vi "Bench_Tests.vi"() -> ()   [LabVIEW 2026]
panel:
  out "cell sum":dbl
  out "limits ok?":bool
  out "results":T1(array[cluster])
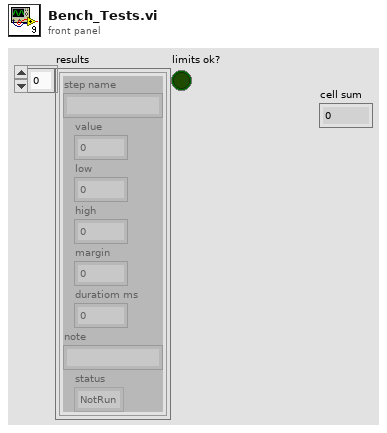
[diagram p1: front panel]
types:
  T1 = cluster{"step name":string, "value":dbl, "low":dbl, "high ":dbl, "margin":dbl, "duratiom ms":dbl, "note":string, "status":enum16{"NotRun", "Pass", "Fail", "Skipped"}}[]
  T2 = cluster{"iso low":dbl, "iso high":dbl, "cell low":dbl, "cell high":dbl, "dv low":dbl, "dv high":dbl, "pack low":dbl, "pack high":dbl}
  T3 = cluster{"step name":string, "value":dbl, "low":dbl, "high ":dbl, "margin":dbl, "duration ms":dbl, "note":string, "status":enum16{"NotRun", "Pass", "Fail", "Skipped"}}[]
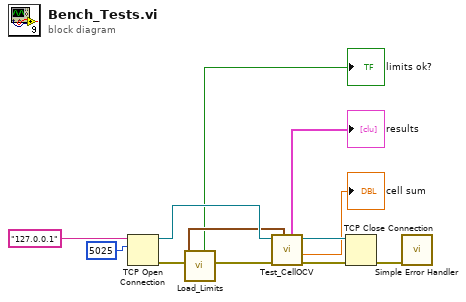
[diagram p0: block diagram]
diagram:
  n1 = TCP Open Connection(address="127.0.0.1", remote port or service name=u16 5025) -> (connection ID=w7:refnum<k5>, error out=w10:errorcluster)  [unwired: 3 in]
  n2 = call "Load_Limits.vi"("error in (no error)"=w10) -> ("error out"=w9:errorcluster, "limits ok?"=→"limits ok?":bool, "Limits"=w5:T2)  [unwired: 7 in, 1 out]
  n3 = call "Test_CellOCV.vi"("Limits"=w5, "error in (no error) 2"=w9, "connection ID 2"=w7) -> ("error out 2"=w8:errorcluster, "cell sum"=→"cell sum":dbl, "connection ID out 2"=w6:refnum<k5>, "results"=→"results":T3)  [unwired: 1 in, 4 out]
  n4 = TCP Close Connection(connection ID=w6, error in (no error)=w8) -> (error out=w2:errorcluster)  [unwired: 1 in, 1 out]
  n5 = call <vilib>:"Simple Error Handler.vi"("error in (no error)"=w2) -> ()  [unwired: 4 in, 5 out]
